vi "Move_Daliy_Folder.vi"(9 "目標資料夾":path=path "C:/ZDX201_報表輸出資料夾/2022_6_25/扭力曲線", 11 "指定鎖螺絲名稱":string) -> ()   [LabVIEW 2019]
panel:
  out "standard output 2":string
  out "concatenated string":string
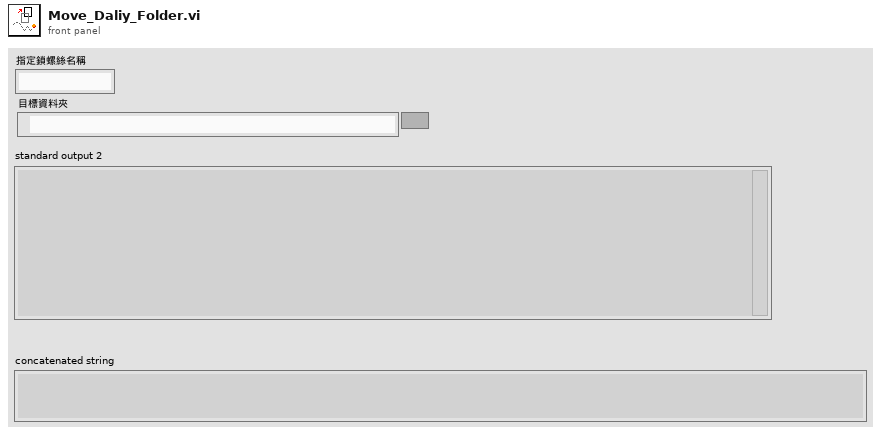
[diagram p1: front panel]
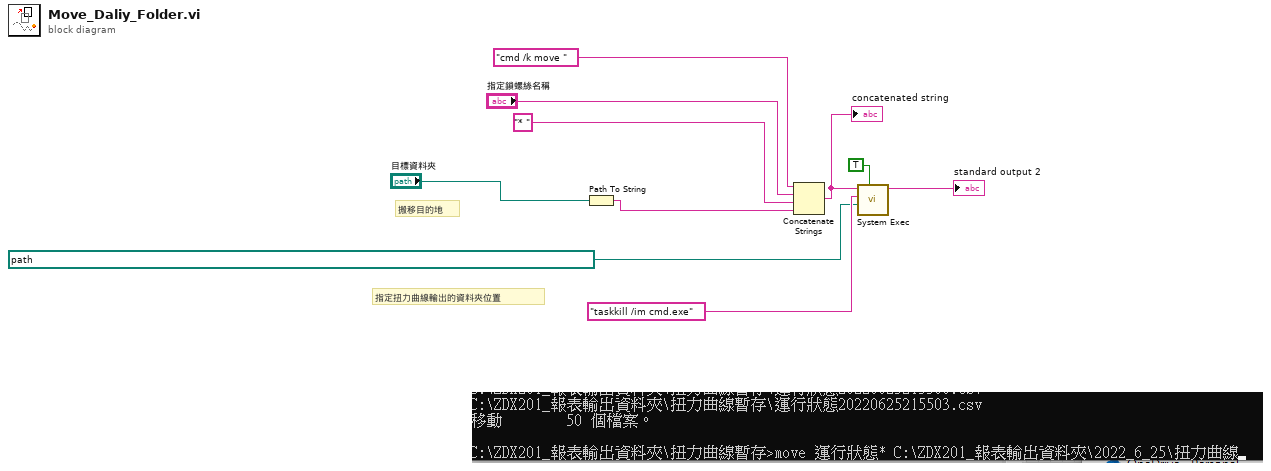
[diagram p0: block diagram]
diagram:
  # "搬移目的地"
  # "指定扭力曲線輸出的資料夾位置"
  n1 = Path To String(path="目標資料夾") -> (string=w1:string)
  n2 = Concatenate Strings("cmd /k move " ("command line"), "指定鎖螺絲名稱", "* " ("string"), w1) -> (w8:string)
  "concatenated string" <- w8
  n3 = call <vilib>:"System Exec.vi"("wait until completion? (T)"=TRUE, "working directory"=path "C:/Users/user/Documents/ESTIC/DataLogger/扭力曲線暫存", "standard input"="taskkill /im cmd.exe", "command line"=w8) -> ("standard output"=→"standard output 2":string)  [unwired: 4 in, 3 out]
